vi "Protected Pointer Error Info.vi"(11 "error":T1) -> (3 "error info":cluster{"code":i32, "description":string})   [LabVIEW 2016, in "Memory Manager.lvlib" / "Protected Pointer.lvclass"]
uses:
  Protected Pointer.lvclass
  Errors.ctl
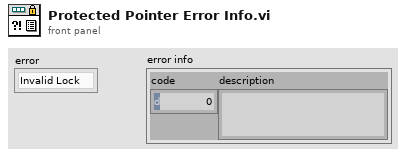
[diagram p1: front panel]
types:
  T1 = typedef "Memory Manager.lvlib/Protected Pointer.lvclass/Errors.ctl" = enum16{"Invalid Lock"}
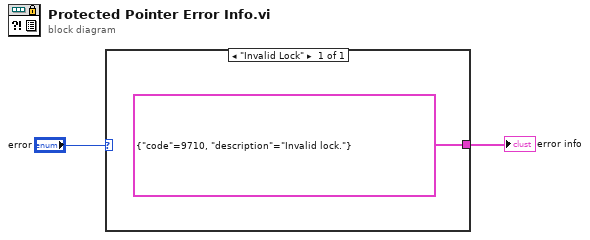
[diagram p0: block diagram]
diagram:
  n1 = case shown="\"Invalid Lock\"" "error" {
    tunnel: [cluster{"code":i32, "description":string} {"code"=9710, "description"="Invalid lock."} ("error info")] -> w1
    frame "Invalid Lock" {
    }
  }
  "error info" <- w1
